vi "peristaltic pump (mLpermin).vi"(4 "State":i16, 5 "Time":dbl format="%.2f", 6 "Sensor Values":dbl[](array[numeric]), 7 "Set Points":dbl[](array[numeric])) -> (0 "required data":T1={"Set Point names"=["flow rate (mL/min)", "Tubing size code"], "required number of setpoints"=2, "required number of sensors"=0, "Sensor names"=[]}, 3 "output value":dbl)   [LabVIEW 2012]
panel:
  in  "pumpflow":dbl[unit][](array[numeric])=[9.549296547316535e-09, 3.342253804929783e-08, 1.2732395447351617e-07, 2.705634032562094e-07, 4.4563384065730255e-07, 6.04788783748884e-07] format="%.3f"
  in  "tubing size":enum16{"13", "14", "16", "25", "17", "18"}(ring)
  # "Enter the correct information for this control code in the required data structure below. Then make the current value default by right clicking on the border of the data structure."
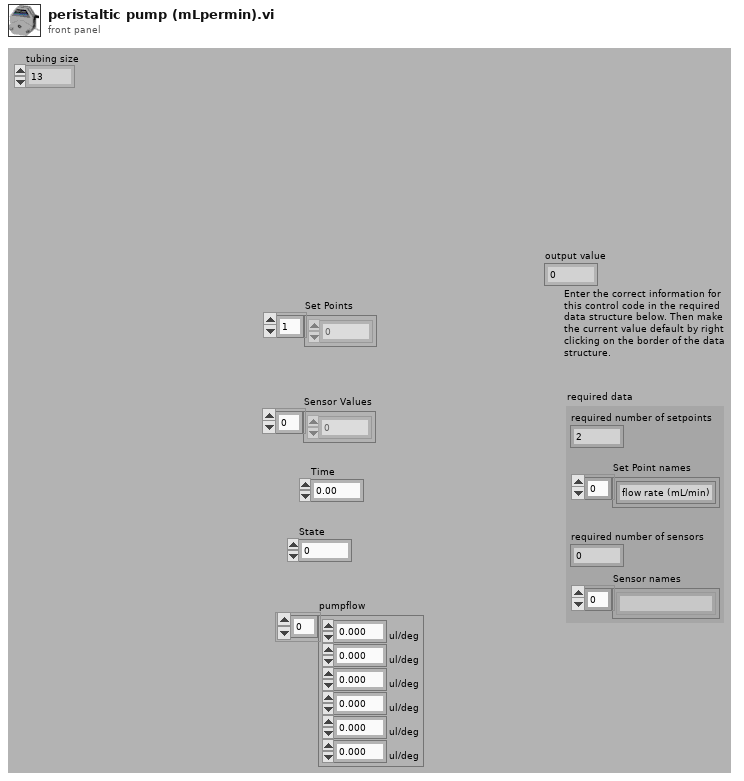
[diagram p1: front panel]
types:
  T1 = cluster{"Set Point names":string[], "required number of setpoints":u8, "required number of sensors":u8, "Sensor names":string[]}
  T2 = cluster{"Set Points[0]":dbl, "Set Points[1]":dbl}
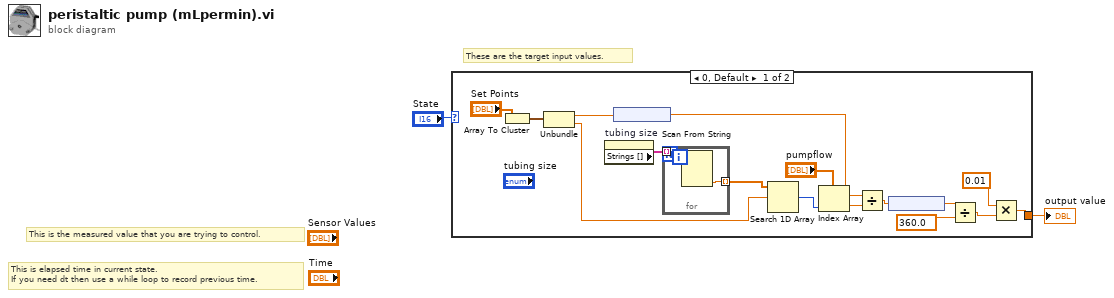
[diagram p0: block diagram]
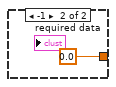
[diagram p2: hidden frame]
diagram:
  # "These are the target input values."
  # "This is the measured value that you are trying to control."
  # "This is elapsed time in current state.\nIf you need dt then use a while loop to record previous time."
  n1 = case shown="0, Default" "State" {
    tunnel: [w12 0.0 ("fraction on")] -> w1
    frame 0, Default {
      n2 = Array To Cluster(array="Set Points") -> (cluster=w18:T2)
      n3 = Unbundle(w18) -> ("Set Points[0]"=w13:dbl, "Set Points[1]"=w3:dbl)
      n4 = property on="tubing size" class="Enum (strict)"() -> ("Strings []"=w14:string[])  [unwired: 2 in, 2 out]
      n5 = node(w13) -> (w4:dbl[unit])
      n6 = for {
        tunnel: w14 -> [w20] mode=indexing
        tunnel: [w19] -> w17 mode=indexing
        n7 = Scan From String(input string=w20) -> (output 1=w19:dbl)  [unwired: 4 in, 3 out]
      }
      n8 = Search 1D Array(1D array=w17, element=w3) -> (index of element=w5:i32)  [unwired: 1 in]
      n9 = Index Array(array="pumpflow", index=w5) -> (element=w10:dbl[unit])
      n10 = Divide(x=w4, y=w10) -> (x/y=w9:dbl[unit])
      n11 = node(w9) -> (w8:dbl)
      n12 = Divide(x=w8, y=360.0) -> (x/y=w6:dbl)
      n13 = Multiply(x=0.01, y=w6) -> (x*y=w12:dbl)
    }
    frame -1 {
    }
  }
  "output value" <- w1
